vi "Tetra_ImonFullTest.vi"(0 "COMPORT":refnum<visa-resource-name>="COM3", 11 "error in (no error)":errorcluster, 12 "Open Ser(t)":bool=TRUE, 13 "Clear errors in(t)":bool=TRUE, 14 "Close Ser(t)":bool=TRUE) -> (1 "rdiv(i)":dbl[](array[numeric])=[0.496, 0.123, 0.534, 0.268, 1.131, 1.12], 2 "rdiv(v)":dbl[](array[numeric])=[3.448, 5.448, 2.832, 2.896, 2.352, 1.448], 3 "Results":string="Name      sw3p6     sw5p5     sw2p8a    sw2p8b    sw2p4     sw1p4     \r\nrdv(v)    3.448     5.448     2.832     2.896     2.352     1.448     \r\nvolt_lsl  3.400     5.400     2.750     2.750     2.300     1.300     \r\nvolt_hsl  3.700     5.600     2.950     2.950     2.600     1.600     \r\nP/F       PASS      PASS      PASS      PASS      PASS      PASS      \r\nrdv(i)    0.496     0.123     0.534     0.268     1.131     1.120     \r\ncurr_lsl  0.200     0.100     0.300     0.200     1.000     0.700     \r\ncurr_hsl  0.500     0.200     0.800     0.400     1.500     1.500     \r\nP/F       PASS      PASS      PASS      PASS      PASS      PASS      \r\n", 4 "comport":refnum<visa-resource-name>="COM3", 6 "Fail?(t)":bool, 8 "Names":string[](array[string])=["sw3p6", "sw5p5", "sw2p8a", "sw2p8b", "sw2p4", "sw1p4"], 15 "error out":errorcluster)   [LabVIEW 2018]
panel:
  out "Result_ary":string[][](array[string])=[["Name", "sw3p6", "sw5p5", "sw2p8a", "sw2p8b", "sw2p4", "sw1p4"], ["rdv(v)", "3.448", "5.448", "2.832", "2.896", "2.352", "1.448"], ["volt_lsl", "3.400", "5.400", "2.750", "2.750", "2.300", "1.300"], ["volt_hsl", "3.700", "5.600", "2.950", "2.950", "2.600", "1.600"], ["P/F", "PASS", "PASS", "PASS", "PASS", "PASS", "PASS"], ["rdv(i)", "0.496", "0.123", "0.534", "0.268", "1.131", "1.120"], ["curr_lsl", "0.200", "0.100", "0.300", "0.200", "1.000", "0.700"], ["curr_hsl", "0.500", "0.200", "0.800", "0.400", "1.500", "1.500"], ["P/F", "PASS", "PASS", "PASS", "PASS", "PASS", "PASS"]]
  in  "Tab Control":enum32{"Page 1", "Comms", "Diagram"}(tab)
  in  "Meas_Limits":bool=TRUE
  in  "rdiv(v)_lim":dbl[][](array[numeric])=[[3.4, 5.4, 2.75, 2.75, 2.3, 1.3], [3.7, 5.6, 2.95, 2.95, 2.6, 1.6]]
  in  "rdiv(i)_lim":dbl[][](array[numeric])=[[0.2, 0.1, 0.25, 0.18, 1.0, 0.7], [0.5, 0.2, 0.8, 0.4, 1.5, 1.5]]
  out "Result  0|1[PASS/FAIL]: dcv(7b) dci(7b)":string="1  111111 111111"
  out "sw_dcv_good":bool[](array[boolean])=[TRUE, TRUE, TRUE, TRUE, TRUE, TRUE]
  out "sw_dci_good":bool[](array[boolean])=[TRUE, TRUE, TRUE, TRUE, TRUE, TRUE]
  out "concatenated string 2":string="rdiv\r\n0)  sw3p6:   496 mA  3448 mV\r\n1)  sw5p5:   123 mA  5448 mV\r\n2) sw2p8a:   534 mA  2832 mV\r\n3) sw2p8b:   268 mA  2896 mV\r\n4)  sw2p4:  1131 mA  2352 mV\r\n5)  sw1p4:  1120 mA  1448 mV\r\n>"
  # "This vi will query the on board i2c current monitors on Tetra WAM rev B0.5 via FPGA"
  # "Readback"
  # "Set Limits"
  # "LSL"
  # "HSL"
  # "LSL"
  # "HSL"
  # "5083549_Release_B_05.PDF"
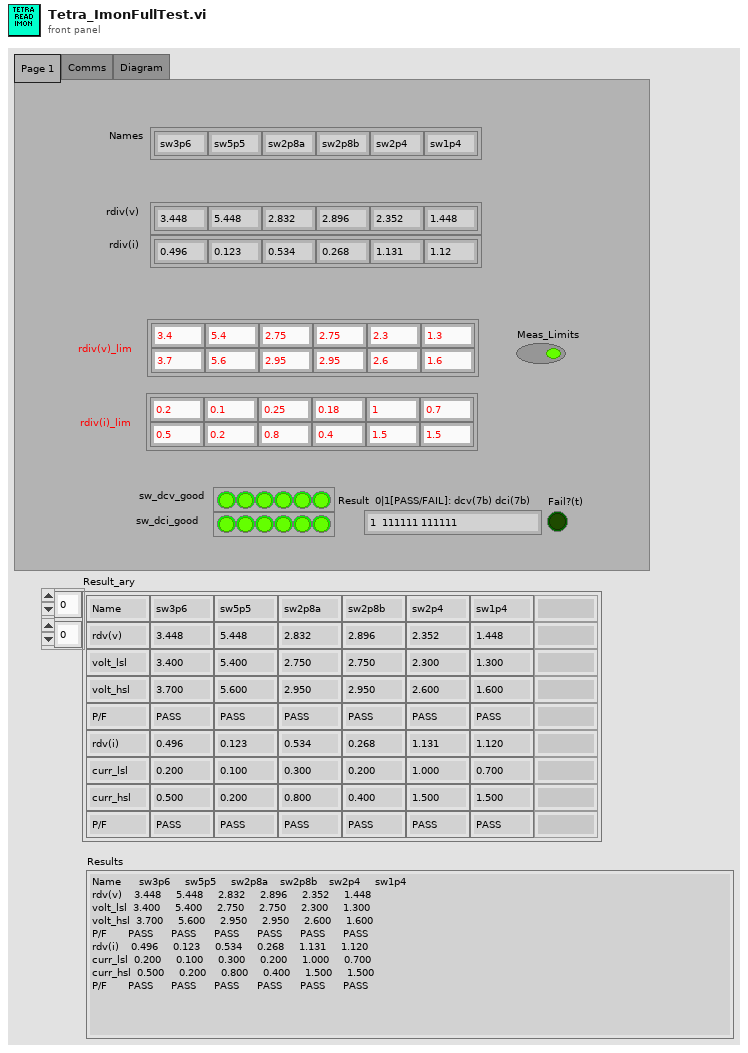
[diagram p1: front panel]
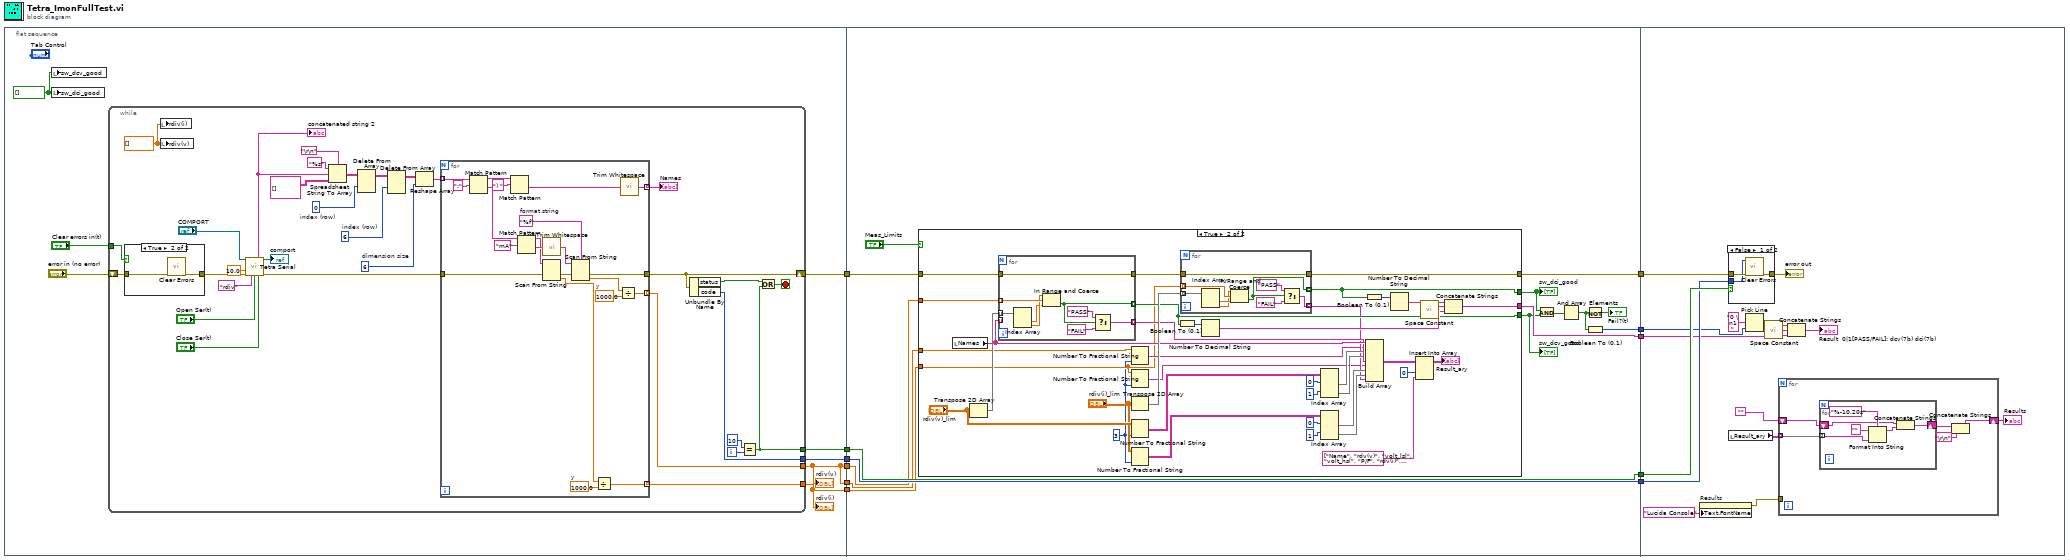
[diagram p0: block diagram]
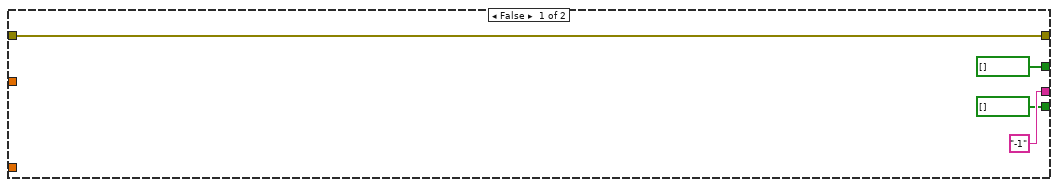
[diagram p3: hidden frame]
diagram:
  n1 = flat-sequence {
    tunnel: [w17] -> w11
    tunnel: [w16] -> w10
    tunnel: [w15] -> w9
    tunnel: [w14] -> w8
    tunnel: [w12] -> w7
    tunnel: [w12] -> w1
    tunnel: w11 -> [w90]
    tunnel: w10 -> [w86]
    tunnel: w9 -> [w89]
    tunnel: w8 -> [w88]
    tunnel: w7 -> [w87]
    tunnel: [w90] -> w6
    tunnel: [w85] -> w5
    tunnel: [w89] -> w4
    tunnel: [w84] -> w3
    tunnel: [w80] -> w2
    tunnel: w1 -> [w76]
    tunnel: w6 -> [w164]
    tunnel: w5 -> [w163]
    tunnel: w4 -> [w162]
    tunnel: w3 -> [w161]
    tunnel: w2 -> [w157]
    frame #0 {
      w13 = bool[] [] ("sw_dci_good")
      n2 = local write "sw_dcv_good"(w13) -> ()
      n3 = local write "sw_dci_good"(w13) -> ()
      n4 = while {
        tunnel: [w51] -> w12
        tunnel: [w50] -> w14
        tunnel: "Clear errors in(t)" -> [w47]
        shift-right: [w29] -> w16
        shift-left: "error in (no error)" -> [w48]
        tunnel: [w26] -> w17
        tunnel: [w25] -> w15
        i -> [w28]
        stop <- w30 stop-if-true
        w35 = 6  # dimension size
        w37 = 6  # index (row)
        w39 = 0  # index (row)
        w45 = dbl[] []
        n5 = case shown="True" w47 {
          tunnel: [w73 w75] -> w46
          tunnel: w48 -> [w73 w74]
          frame False {
          }
          frame True {
            n6 = call <vilib>:"Clear Errors.vi"("error in (no error)"=w74) -> ("error out"=w75:errorcluster)  [unwired: 5 in, 1 out]
          }
        }
        n7 = local write "rdiv(i)"(w45) -> ()
        n8 = local write "rdiv(v)"(w45) -> ()
        n9 = call "Tetra Serial.vi"("COMPORT"="COMPORT", "Timeout(s)"=10.0, "error in (no error)"=w46, "Command"="rdiv", "Open Ser(t)"="Open Ser(t)", "Close Ser(t)"="Close Ser(t)") -> ("output"=w32:string, "comport"=→"comport":refnum<visa-resource-name>, "error out"=w31:errorcluster)  [unwired: 5 in, 2 out]
        "concatenated string 2" <- w32
        n10 = Spreadsheet String To Array(delimiter (Tab)="\r\n", format string="%s", spreadsheet string=w32, array type (2D Dbl)=string[][] []) -> (array=w40:string[][])
        n11 = Delete From Array(array=w40, index (row)=w39) -> (array with subset deleted=w38:string[][])  [unwired: 2 in, 1 out]
        n12 = Delete From Array(array=w38, index (row)=w37) -> (array with subset deleted=w36:string[][])  [unwired: 2 in, 1 out]
        n13 = Reshape Array(w36, w35) -> (w34:string[])
        n14 = for {
          tunnel: w34 -> [w72] mode=indexing
          tunnel: [w63] -> w51 mode=indexing
          tunnel: [w60] -> w50 mode=indexing
          tunnel: [w56] -> w29
          tunnel: w31 -> [w58]
          tunnel: [w52] -> w22 mode=indexing
          w64 = 1000.0  # y
          w66 = 1000.0  # y
          w68 = "%f"  # format string
          n15 = Match Pattern(string=w72, regular expression=":") -> (before substring=w55:string, after substring=w67:string)  [unwired: 1 in, 2 out]
          n16 = Match Pattern(string=w55, regular expression=") ") -> (after substring=w53:string)  [unwired: 1 in, 3 out]
          n17 = Match Pattern(string=w67, regular expression="mA") -> (before substring=w59:string, after substring=w65:string)  [unwired: 1 in, 2 out]
          n18 = call <vilib>:"Trim Whitespace.vi"("string"=w65) -> ("trimmed string"=w62:string)  [unwired: 1 in]
          n19 = Scan From String(input string=w59, error in=w58) -> (error out=w57:errorcluster, output 1=w61:dbl)  [unwired: 3 in, 2 out]
          n20 = Scan From String(format string=w68, input string=w62, error in=w57) -> (error out=w56:errorcluster, output 1=w69:dbl)  [unwired: 2 in, 2 out]
          n21 = Divide(x=w61, y=w64) -> (x/y=w60:dbl)
          n22 = Divide(x=w69, y=w66) -> (x/y=w63:dbl)
          n23 = call <vilib>:"Trim Whitespace.vi"("string"=w53) -> ("trimmed string"=w52:string)  [unwired: 1 in]
        }
        "Names" <- w22
        n24 = Unbundle By Name(w29) -> ("status"=w20:bool, "code"=w25:i32)
        n25 = Equal?(x=10, y=w28) -> (x = y?=w26:bool)
        n26 = Or(x=w20, y=w26) -> (x .or. y?=w30:bool)
      }
      "rdiv(v)" <- w12
      "rdiv(i)" <- w14
    }
    frame #1 {
      n27 = case shown="True" "Meas_Limits" {
        tunnel: w88 -> [_ w101]
        tunnel: w87 -> [_ w131]
        tunnel: w86 -> [w94 w129]
        tunnel: [w94 w127] -> w85
        tunnel: ["-1" w121] -> w84
        tunnel: [bool[] [] w120] -> w82
        tunnel: [bool[] [] w119] -> w81
        tunnel: w76 -> [_ w103]
        frame False {
        }
        frame True {
          w95 = i16 3 ("precision (6)")
          n28 = local read "Names"() -> (w118:string[])
          n29 = Transpose 2D Array(2D array="rdiv(v)_lim") -> (transposed array=w132:dbl[][])
          n30 = for {
            tunnel: [w136] -> w119 mode=indexing
            tunnel: w132 -> [w141] mode=indexing
            tunnel: w131 -> [w140] mode=indexing
            tunnel: w118 -> [_] mode=indexing
            tunnel: w129 -> [w137]
            tunnel: [w137] -> w128
            tunnel: [w133] -> w117 mode=indexing
            n31 = Index Array(array=w141) -> (element #1=w138:dbl, element #2=w139:dbl)  [unwired: 2 in]
            n32 = In Range and Coerce(upper limit=w139, x=w140, lower limit=w138) -> (In Range?=w136:bool)  [unwired: 1 out]
            n33 = Select(t="PASS", s=w136, f="FAIL") -> (s? t:f=w133:string)
          }
          n34 = Number To Fractional String(number=w103, precision (6)=w95) -> (F-format string=w102:string[])  [unwired: 2 in]
          n35 = Number To Fractional String(number=w101, precision (6)=w95) -> (F-format string=w100:string[])  [unwired: 2 in]
          n36 = Transpose 2D Array(2D array="rdiv(i)_lim") -> (transposed array=w130:dbl[][])
          n37 = Number To Fractional String(number="rdiv(v)_lim", precision (6)=w95) -> (F-format string=w113:string[][])  [unwired: 2 in]
          n38 = Number To Fractional String(number="rdiv(i)_lim", precision (6)=w95) -> (F-format string=w110:string[][])  [unwired: 2 in]
          n39 = Boolean To (0,1)(Boolean=w119) -> (0, 1=w123:i16[])
          n40 = for {
            tunnel: [w143] -> w120 mode=indexing
            tunnel: w101 -> [w150] mode=indexing
            tunnel: w130 -> [w147] mode=indexing
            tunnel: w128 -> [w146]
            tunnel: [w146] -> w127
            tunnel: [w142] -> w104 mode=indexing
            n41 = Index Array(array=w147) -> (element #1=w149:dbl, element #2=w148:dbl)  [unwired: 2 in]
            n42 = In Range and Coerce(upper limit=w148, x=w150, lower limit=w149) -> (In Range?=w143:bool)  [unwired: 1 out]
            n43 = Select(t="PASS", s=w143, f="FAIL") -> (s? t:f=w142:string)
          }
          n44 = Number To Decimal String(number=w123) -> (decimal integer string=w125:string[])  [unwired: 1 in]
          n45 = Index Array(array=w113, index (row) #1=0 ("index (row)"), index (row) #2=1 ("index (row)")) -> (element #1=w112:string[], element #2=w111:string[])  [unwired: 2 in]
          n46 = Index Array(array=w110, index (row) #1=0 ("index (row)"), index (row) #2=1 ("index (row)")) -> (element #1=w106:string[], element #2=w105:string[])  [unwired: 2 in]
          n47 = Boolean To (0,1)(Boolean=w120) -> (0, 1=w122:i16[])
          n48 = Build Array(w118, w102, w112, w111, w117, w100, w106, w105, w104) -> (w98:string[][])
          n49 = Number To Decimal String(number=w122) -> (decimal integer string=w124:string[])  [unwired: 1 in]
          n50 = Insert Into Array(array=w98, index (col)=0 ("disabled index (col)"), new element=string[] ["Name", "rdv(v)", "volt_lsl", "volt_hsl", "P/F", "rdv(i)", "curr_lsl", "curr_hsl", "P/F"] ("new element/subarray")) -> (→"Result_ary":string[][])  [unwired: 1 in]
          n51 = call <vilib>:"Space Constant.vi"() -> ("String"=w126:string)
          n52 = Concatenate Strings(w124, w126, w125) -> (w121:string)
        }
      }
      "sw_dci_good" <- w82
      "sw_dcv_good" <- w81
      n53 = And(x=w82, y=w81) -> (x .and. y?=w79:bool[])
      n54 = And Array Elements(Boolean array=w79) -> (logical AND=w78:bool)
      n55 = Not(x=w78) -> (.not. x?=→"Fail?(t)":bool)
      n56 = Boolean To (0,1)(Boolean=w78) -> (0, 1=w80:i16)
    }
    frame #2 {
      n57 = property on="Results" class="Str"("Text.FontName"="Lucida Console" ("Text.Font:Name")) -> (error out=w151:errorcluster)  [unwired: 2 in, 1 out]
      n58 = case shown="False" w164 {
        tunnel: w163 -> [w179 w180]
        tunnel: [w178 w180] -> w165
        tunnel: w162 -> [w177 _]
        frame False {
          n59 = call <vilib>:"Clear Errors.vi"("error in (no error)"=w179, "specific error code to clear (0: all)"=w177) -> ("error out"=w178:errorcluster)  [unwired: 4 in, 1 out]
        }
        frame True {
        }
      }
      "error out" <- w165
      n60 = local read "Result_ary"() -> (w155:string[][])
      n61 = Pick Line(multi-line string="0 \n1 ", line index=w157) -> (output string=w156:string)  [unwired: 1 in]
      n62 = call <vilib>:"Space Constant.vi"() -> ("String"=w159:string)
      n63 = for {
        tunnel: w155 -> [w170] mode=indexing
        shift-right: [w168] -> w154
        shift-left: "" -> [w166]
        tunnel: w151 -> [_]
        n64 = for {
          tunnel: w170 -> [w175] mode=indexing
          shift-right: [w173] -> w169
          shift-left: w166 -> [w171]
          n65 = Format Into String(format string="%-10.20s", initial string="", w175) -> (resulting string=w174:string)  [unwired: 1 in, 1 out]
          n66 = Concatenate Strings(w171, w174) -> (w173:string)
        }
        n67 = Concatenate Strings(w169, "\r\n") -> (w168:string)
      }
      "Results" <- w154
      n68 = Concatenate Strings(w156, w159, w161) -> (→"Result  0|1[PASS/FAIL]: dcv(7b) dci(7b)":string)
    }
  }
